vi "Get Write Data.vi"(8 "Multiplication Factor":dbl=1.0, 9 "Sampling information 2":cluster{"Fs":dbl, "#s":dbl}[](array[cluster])=[{"Fs"=10000.0, "#s"=5000.0}, {"Fs"=10000.0, "#s"=5000.0}], 10 "AO Task":refnum<k21>[](array[refnum])=[""], 11 "OSC Configuration":T1(array[cluster])=[[{"Signal Type"=enum."Sine Wave", "DC"=0.0, "Amplitude"=0.01, "frequency"=2.0, "Phase"=0.0}, {"Signal Type"=enum."Sine Wave", "DC"=0.0, "Amplitude"=0.01, "frequency"=2.0, "Phase"=0.0}], [{"Signal Type"=enum."Sine Wave", "DC"=0.0, "Amplitude"=0.01, "frequency"=2.0, "Phase"=0.0}, {"Signal Type"=enum."Sine Wave", "DC"=0.0, "Amplitude"=0.01, "frequency"=2.0, "Phase"=0.0}]] {"frequency" step=0.001 format="%.3p"; "Amplitude" format="%0.2p"; "DC" min=-0.99 max=0.99 format="%.2p"}) -> (3 "Data":waveform(dbl)[][](array[waveform]))   [LabVIEW 2013]
uses:
  <vilib>/measure/NI_MABase.lvlib
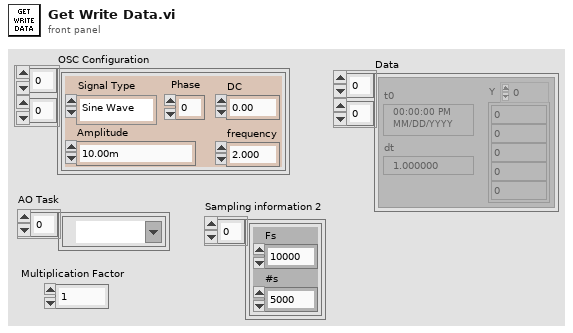
[diagram p1: front panel]
types:
  T1 = cluster{"Signal Type":enum16{"Sine Wave", "Triangle Wave", "Square Wave", "Sawtooth Wave"}, "DC":dbl, "Amplitude":dbl, "frequency":dbl, "Phase":dbl}[][]
  T2 = cluster{"Signal Type":enum16{"Sine Wave", "Triangle Wave", "Square Wave", "Sawtooth Wave"}, "DC":dbl, "Amplitude":dbl, "frequency":dbl, "Phase":dbl}
  T3 = enum16{"Sine Wave", "Triangle Wave", "Square Wave", "Sawtooth Wave"}
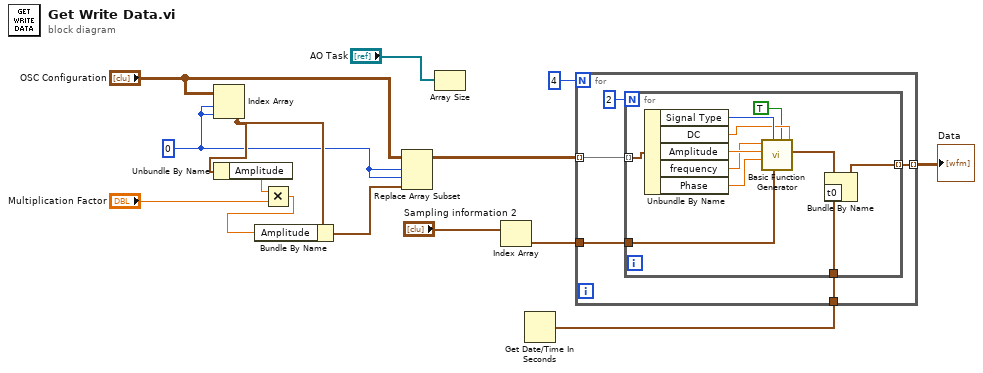
[diagram p0: block diagram]
diagram:
  w10 = 0 ("index")
  n1 = Index Array(array="OSC Configuration", index (row)=w10, index (col)=w10) -> (element=w14:T2)
  n2 = Unbundle By Name(w14) -> ("Amplitude"=w13:dbl)
  n3 = Multiply(x=w13, y="Multiplication Factor") -> (x*y=w12:dbl)
  n4 = Bundle By Name(cluster=w14, "Amplitude"=w12) -> (w11:T2)
  n5 = Replace Array Subset(array="OSC Configuration", new element=w11, index (row)=w10, index (col)=w10) -> (w8:T1)
  n6 = Array Size(array="AO Task") -> ()  [unwired: 1 out]
  n7 = Index Array(array="Sampling information 2") -> (element=w2:cluster{"Fs":dbl, "#s":dbl})  [unwired: 1 in]
  n8 = Get Date/Time In Seconds() -> (seconds since 1Jan1904=w1:timestamp)
  n9 = for {
    N: 4 -> [_]
    tunnel: [w19] -> w9 mode=indexing
    tunnel: w8 -> [w18] mode=indexing
    tunnel: w2 -> [w16]
    tunnel: w1 -> [w15]
    n10 = for {
      N: 2 -> [_]
      tunnel: w18 -> [w25] mode=indexing
      tunnel: [w20] -> w19 mode=indexing
      tunnel: w16 -> [w23]
      tunnel: w15 -> [w21]
      n11 = Unbundle By Name(w25) -> ("Signal Type"=w30:T3, "DC"=w29:dbl, "Amplitude"=w28:dbl, "frequency"=w27:dbl, "Phase"=w26:dbl)
      n12 = call <vilib>:"Basic Function Generator.vi"("offset"=w29, "reset signal"=TRUE, "sampling info"=w23, "signal type"=w30, "phase"=w26, "amplitude"=w28, "frequency"=w27) -> ("signal out"=w22:waveform(dbl))  [unwired: 2 in, 2 out]
      n13 = Bundle By Name(cluster=w22, "t0"=w21) -> (w20:waveform(dbl))
    }
  }
  "Data" <- w9
